vi "mks946_acquire.vi"(8 "error in":errorcluster) -> (0 "error out":errorcluster)   [LabVIEW 2019]
doc: "Perform the acquisition. Replace the contents of this diagram with calls to acquisition hardware.\n_____\nBased on Delacor QMH Project Template 5.0.0.82."
panel:
  in  "n_pt_max":i32 caption="in plot"
  in  "interval":dbl=0.5 caption="in sec" format="%#_13g"
  out "graph_ch2":T1(graph)
  out "graph_ch1":T1(graph)
  in  "stop":bool
  out "value_ch2":dbl
  out "value_ch1":dbl
  out "measurement time":timestamp
  in  "address":i32=253
  out "visa_out":refnum<visa-resource-name>="COM3"
  in  "visa_in":refnum<visa-resource-name>="COM3"
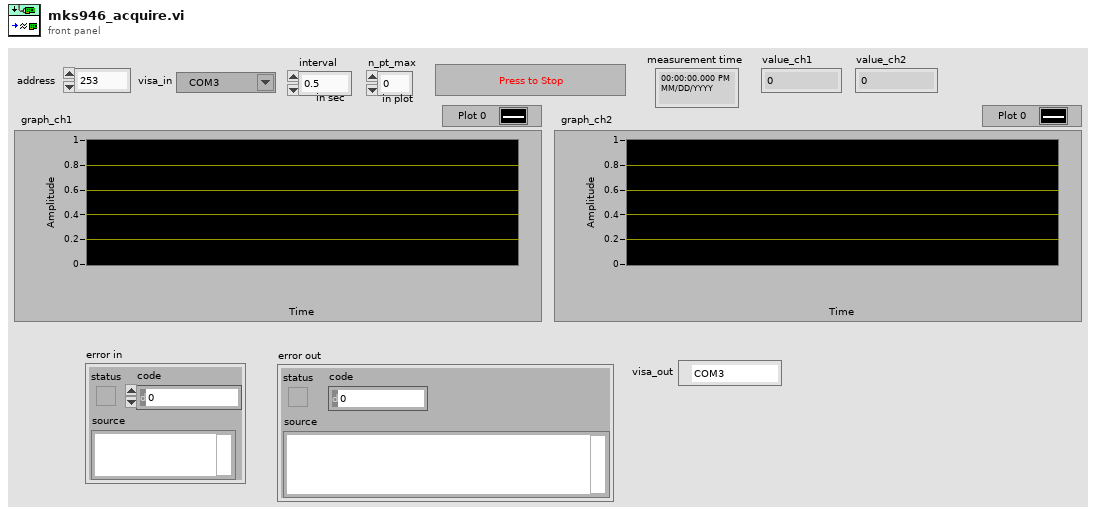
[diagram p1: front panel]
types:
  T1 = cluster{"seconds since 1Jan1904":timestamp, "value":dbl}[]
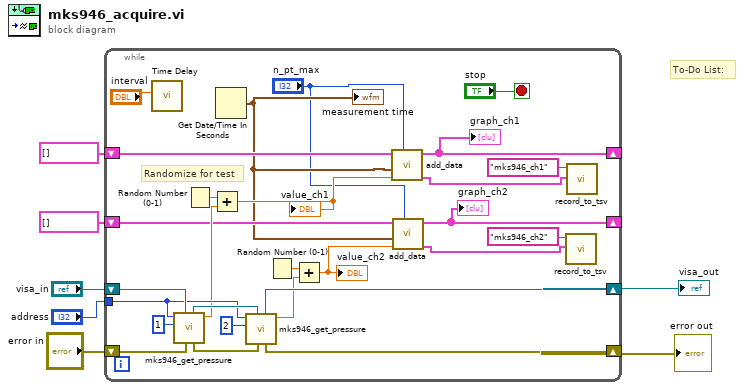
[diagram p0: block diagram]
diagram:
  # "To-Do List:"
  n1 = while {
    tunnel: "address" -> [w27]
    shift-right: [w30] -> w5
    shift-left: "visa_in" -> [w34]
    shift-right: [w26] -> w3
    shift-left: "error in" -> [w32]
    shift-right: [w16] -> _
    shift-left: T1 [] ("graph_ch1") -> [w17]
    shift-right: [w13] -> _
    shift-left: T1 [] ("graph_ch1") -> [w12]
    stop <- "stop" stop-if-true
    # "Randomize for test"
    n2 = call "Time Delay"("Delay Time (s)"="interval") -> ()  [unwired: 10 in, 1 out]
    n3 = call "mks946_get_pressure.vi"("err_in"=w32, "visa_in"=w34, "channel"=1, "address"=w27) -> ("value"=w23:dbl, "err_out"=w29:errorcluster, "visa_out"=w31:refnum<visa-resource-name>)  [unwired: 3 in, 2 out]
    n4 = Random Number (0-1)() -> (number: 0 to 1=w22:dbl)
    n5 = Add(x=w22, y=w23) -> (x+y=w15:dbl)
    "value_ch1" <- w15
    n6 = Get Date/Time In Seconds() -> (seconds since 1Jan1904=w11:timestamp)
    "measurement time" <- w11
    n7 = call "mks946_get_pressure.vi"("err_in"=w29, "visa_in"=w31, "channel"=2, "address"=w27) -> ("value"=w20:dbl, "err_out"=w26:errorcluster, "visa_out"=w30:refnum<visa-resource-name>)  [unwired: 3 in, 2 out]
    n8 = Random Number (0-1)() -> (number: 0 to 1=w21:dbl)
    n9 = Add(x=w21, y=w20) -> (x+y=w10:dbl)
    "value_ch2" <- w10
    n10 = call "add_data.vi"("n_max"="n_pt_max", "value"=w15, "timestamp"=w11, "array_in"=w17) -> ("cluster_out"=w14:cluster{"timestamp":timestamp, "value":dbl}, "array_out"=w16:T1)  [unwired: 6 in]
    "graph_ch1" <- w16
    n11 = call "add_data.vi"("n_max"="n_pt_max", "value"=w10, "timestamp"=w11, "array_in"=w12) -> ("cluster_out"=w9:cluster{"timestamp":timestamp, "value":dbl}, "array_out"=w13:T1)  [unwired: 6 in]
    "graph_ch2" <- w13
    n12 = call "record_to_tsv.vi"("cluster"=w9, "name"="mks946_ch2") -> ()  [unwired: 10 in]
    n13 = call "record_to_tsv.vi"("cluster"=w14, "name"="mks946_ch1") -> ()  [unwired: 10 in]
  }
  "error out" <- w3
  "visa_out" <- w5
